vi "G8uCharTrace_v1_sub.vi"(0 "Macros":i32[](array[numeric]), 1 "bin time (ns)":i32=1000) -> (2 "error":bool, 3 "Trace Length":i32=5016644, 4 "G1-G8":sgl[](array[numeric])=[1.6120762, 1.4506032, 1.3552333, 1.2686939, 1.1945174, 1.2038525, 1.1705487, 1.0706373] format="%.6f")   [LabVIEW 2009]
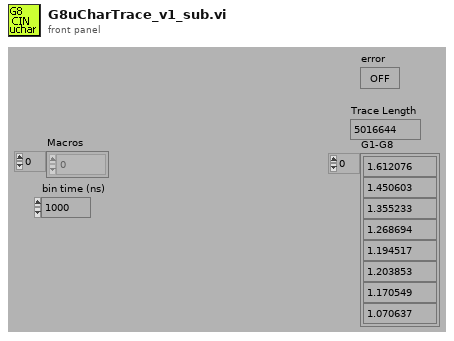
[diagram p1: front panel]
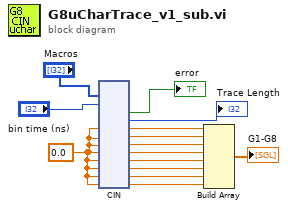
[diagram p0: block diagram]
diagram:
  w9 = sgl 0.0
  n1 = cin("Macros", "bin time (ns)", w9, w9, w9, w9, w9, w9, w9, w9) -> (→"error":bool, →"Trace Length":i32, w8:sgl, w7:sgl, w6:sgl, w5:sgl, w4:sgl, w3:sgl, w2:sgl, w1:sgl)  [unwired: 4 in]
  n2 = Build Array(w8, w7, w6, w5, w4, w3, w2, w1) -> (→"G1-G8":sgl[])
